vi "download file.vi"(8 "error in (no error)":errorcluster, 11 "远端地址":string="/UP/OneStation/V4/一体化微型水质监测站.zip") -> (0 "error out":errorcluster, 3 "local file path":path caption="本地文件路径")   [LabVIEW 2016, in "数据传输系统-03.lvlib" / "update.lvlib"]
uses:
  update.lvlib
  <vilib>/WebDAVClient/Advanced/Multi Event/Request Status.ctl
  WebDAV client/WebDAV client.lvclass
  <vilib>/WebDAVClient/NI_WebDAV.lvlib
panel:
  out "request status":T1
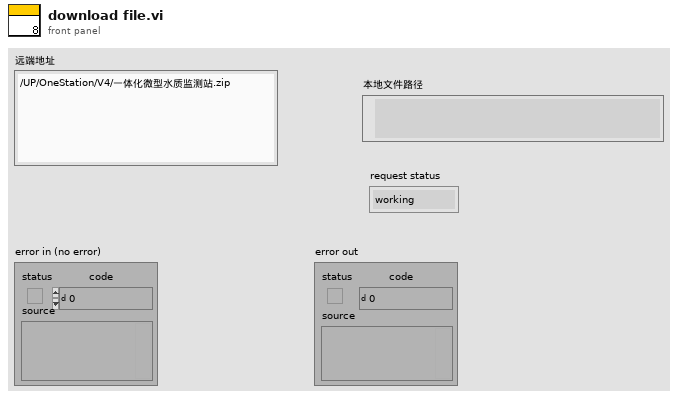
[diagram p1: front panel]
types:
  T1 = typedef "NI_WebDAV.lvlib/Request Status.ctl" = enum16{"working", "complete", "aborted", "timeout", "error"}
  T2 = cluster{"host uri prefix":string, "username":string, "password":string}
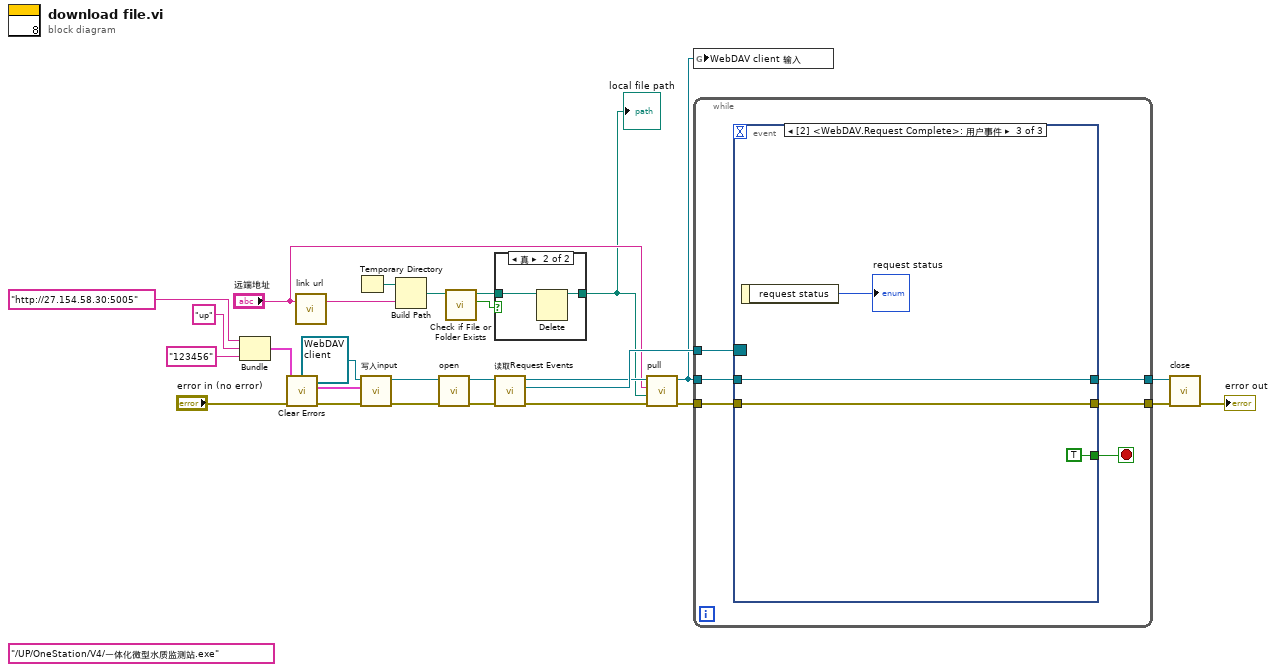
[diagram p0: block diagram]
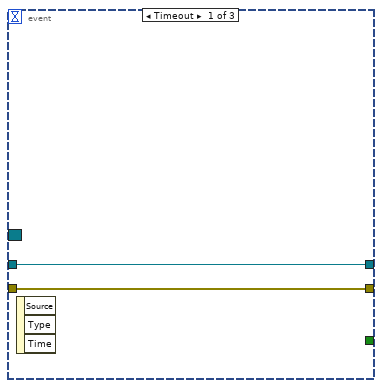
[diagram p3: hidden frame]
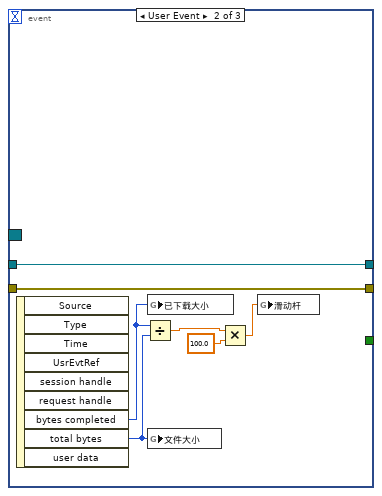
[diagram p4: hidden frame]
diagram:
  (unwired) "/UP/OneStation/V4/一体化微型水质监测站.exe" ("更新包远端地址")
  n1 = Bundle("host uri prefix"="http://27.154.58.30:5005", "username"="up", "password"="123456") -> (w21:T2)  [unwired: 1 in]
  n2 = call <vilib>:"Clear Errors.vi"("error in (no error)"="error in (no error)") -> ("error out"=w1:errorcluster)  [unwired: 5 in, 1 out]
  n3 = call "link url.vi"("远端地址"="远端地址") -> ("file name"=w3:string)  [unwired: 17 in, 1 out]
  n4 = Temporary Directory() -> (w7:path)
  n5 = call-dynamic "写入input.vi"("error in (no error)"=w1, "input"=w21, "WebDAV client输入"=refnum<class "WebDAV client.lvclass"> refnum ("update.lvlib:WebDAV client.lvclass")) -> ("error out"=w20:errorcluster, "WebDAV client输出"=w22:refnum<class "WebDAV client.lvclass">)  [unwired: 7 in]
  n6 = Build Path(base path=w7, name or relative path=w3) -> (appended path=w6:path)
  n7 = call-dynamic "open.vi"("error in (no error)"=w20, "WebDAV client 输入"=w22) -> ("error out"=w19:errorcluster, "WebDAV client 输出"=w18:refnum<class "WebDAV client.lvclass">)  [unwired: 8 in]
  n8 = call <vilib>:"Check if File or Folder Exists.vi"("path"=w6) -> ("file or folder exists?"=w4:bool, "dup path"=w5:path)  [unwired: 8 in, 1 out]
  n9 = case shown="真" w4 {
    tunnel: w5 -> [w27 w29]
    tunnel: [w27 w28] -> w2
    frame False {
    }
    frame True {
      n10 = Delete(path (use dialog)=w29) -> (deleted path=w28:path)  [unwired: 4 in, 2 out]
    }
  }
  "local file path" <- w2
  n11 = call-dynamic "读取Request Events.vi"("error in (no error)"=w19, "WebDAV client输入"=w18) -> ("error out"=w10:errorcluster, "Request Events"=w16:refnum<event-registration>, "WebDAV client输出"=w12:refnum<class "WebDAV client.lvclass">)  [unwired: 7 in]
  n12 = call-dynamic "pull.vi"("error in (no error)"=w10, "local file path"=w2, "更新包远端地址"="远端地址", "WebDAV client 输入"=w12) -> ("error out"=w9:errorcluster, "WebDAV client 输出"=w11:refnum<class "WebDAV client.lvclass">)  [unwired: 6 in]
  n13 = global write "更新全局变量.vi" "WebDAV client 输入"(w11) -> ()
  n14 = while {
    tunnel: w16 -> [w35]
    tunnel: w11 -> [w34]
    tunnel: [w32] -> w15
    tunnel: [w31] -> w14
    tunnel: w9 -> [w30]
    stop <- w33 stop-if-true
    n15 = event shown="[2] <WebDAV.Request Complete>: 用户事件" {
      selector: w35 -> [_ _ _]
      dyn-events: _ -> [_ _ _]
      timeout: _ -> [_ _ _]
      tunnel: w34 -> [w37 w39 w47]
      tunnel: [_ _ TRUE] -> w33
      tunnel: [w37 w39 w47] -> w32
      tunnel: [w36 w38 w46] -> w31
      tunnel: w30 -> [w36 w38 w46]
      event Timeout {
        n16 = event-data() -> ()  [unwired: 1 in, 3 out]
      }
      event User Event {
        n17 = event-data() -> ("bytes completed"=w41:u64, "total bytes"=w42:u64)  [unwired: 1 in, 7 out]
        n18 = Divide(x=w41, y=w42) -> (x/y=w43:dbl)
        n19 = global write "更新全局变量.vi" "已下载大小"(w41) -> ()
        n20 = global write "更新全局变量.vi" "文件大小"(w42) -> ()
        n21 = Multiply(x=w43, y=100.0) -> (x*y=w40:dbl)
        n22 = global write "更新全局变量.vi" "滑动杆"(w40) -> ()
      }
      event User Event {
        n23 = event-data() -> ("request status"=→"request status":T1)  [unwired: 1 in]
      }
    }
  }
  n24 = call-dynamic "close.vi"("error in (no error)"=w14, "WebDAV client 输入"=w15) -> ("error out"=→"error out":errorcluster)  [unwired: 8 in, 1 out]
